vi "server_pos_indicator_v2.vi"(5 "reset":bool, 7 "rough":bool, 8 "error in":errorcluster, 10 "yc":dbl, 11 "xc":dbl) -> (0 "error out":errorcluster)   [LabVIEW 2014]
panel:
  out "resulting string":string
  out "rough Array":bool[](array[boolean])
  out "rough_num":i32
  out "size(s)":i32
  out "output array":T1(array[cluster])
  out "position":picture
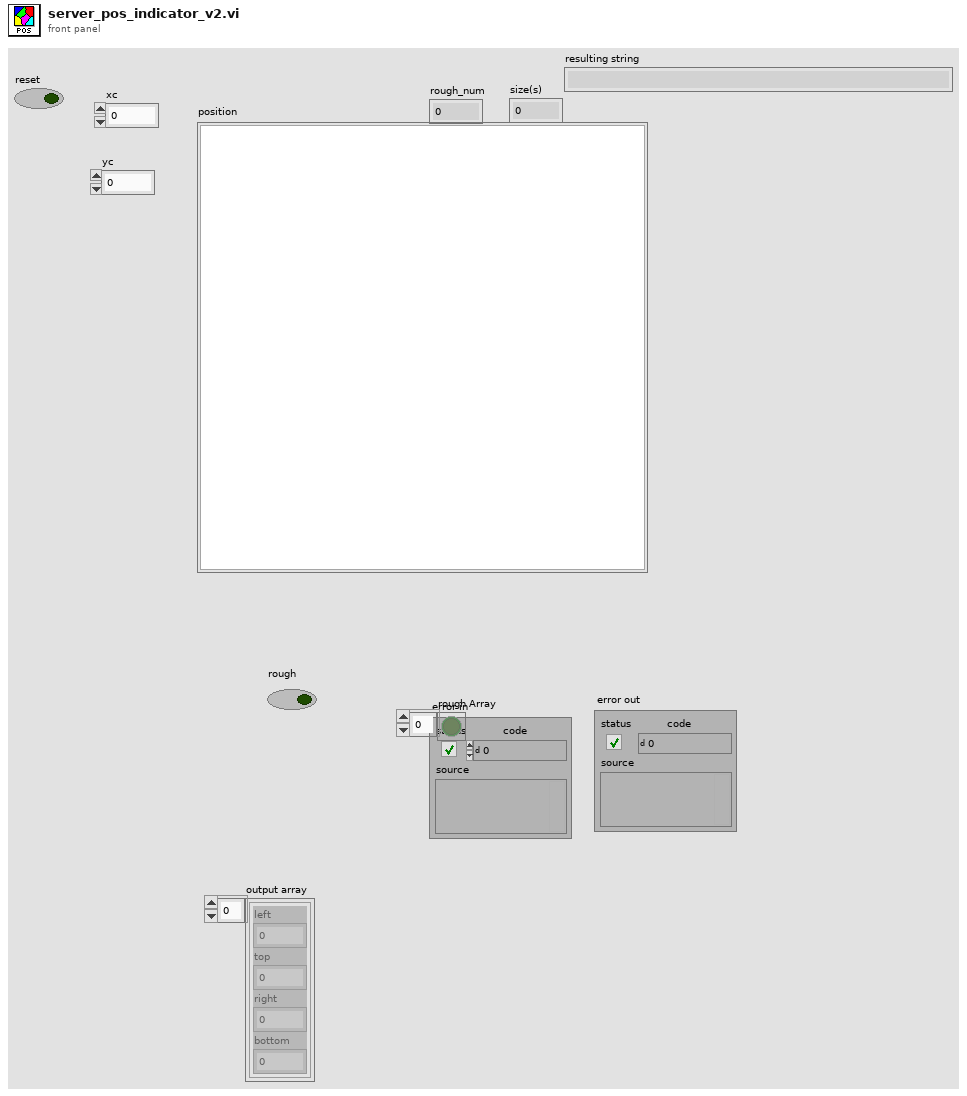
[diagram p1: front panel]
types:
  T1 = cluster{"left":i16, "top":i16, "right":i16, "bottom":i16}[]
  T2 = cluster{"left":i16, "top":i16, "right":i16, "bottom":i16}
  T3 = cluster{"horizontal":enum16{"left", "center", "right"}, "vertical":enum16{"top", "center", "bottom"}}
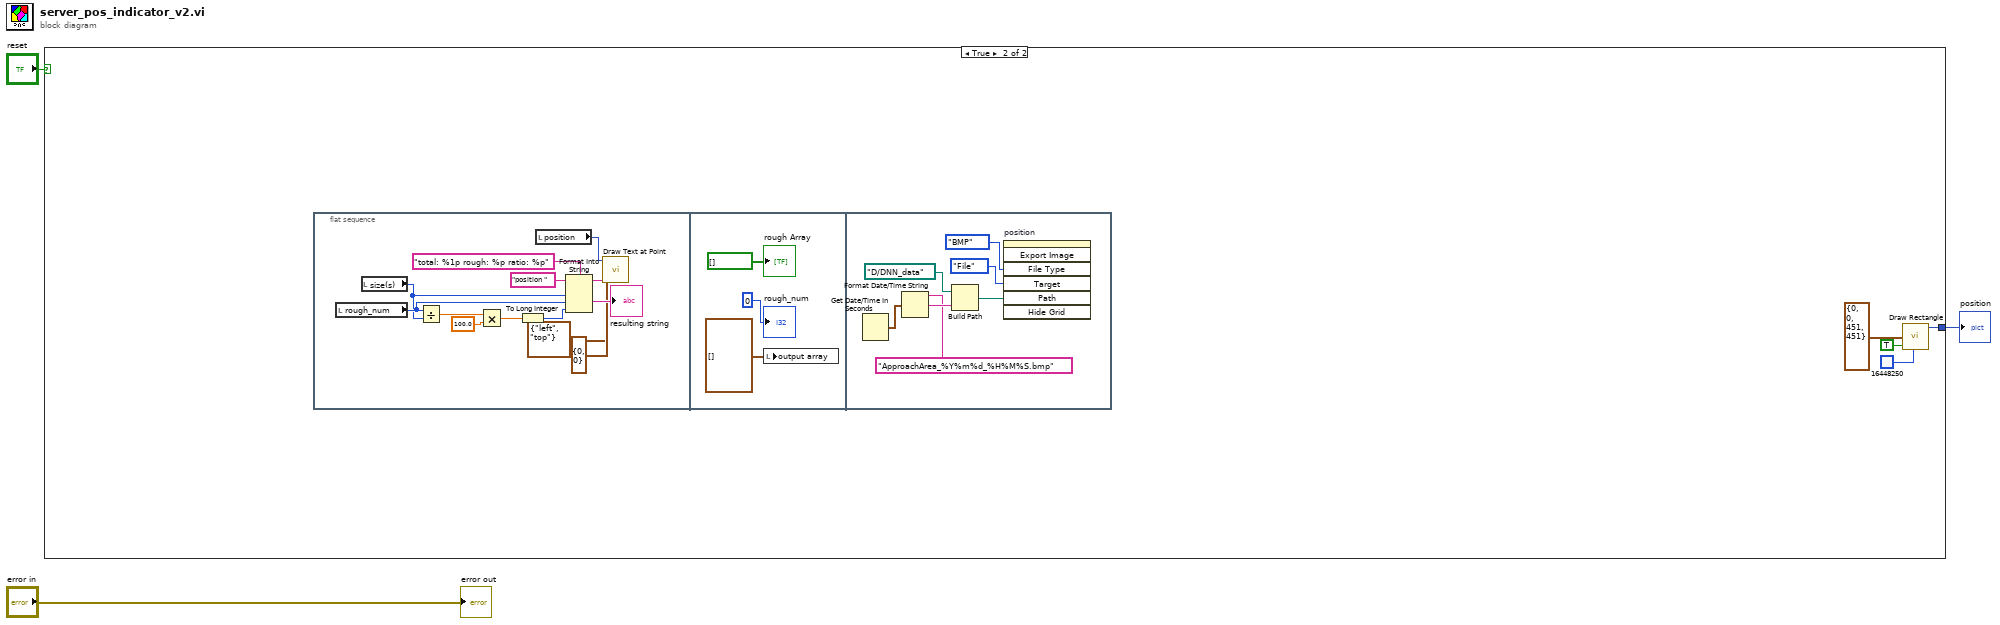
[diagram p0: block diagram]
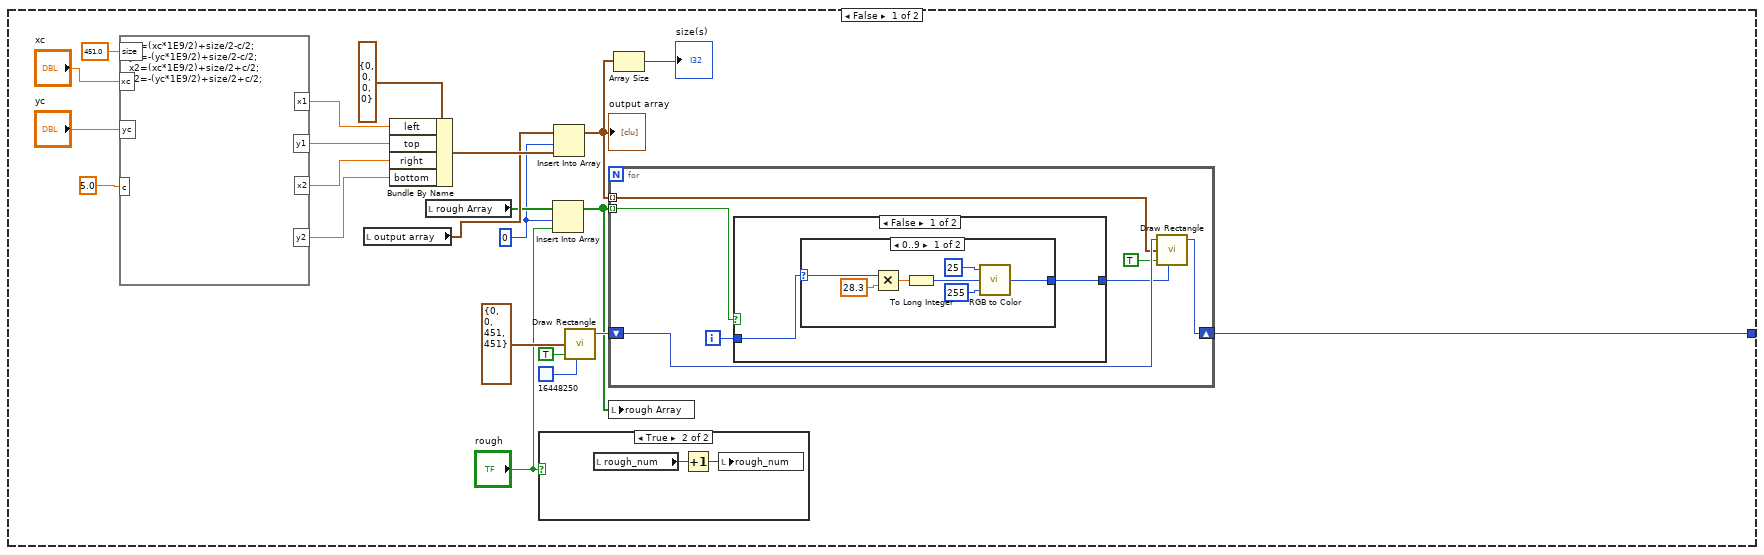
[diagram p2: hidden frame]
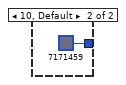
[diagram p4: hidden frame]
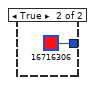
[diagram p5: hidden frame]
diagram:
  n1 = case shown="True" "reset" {
    tunnel: [w22 w46] -> w2
    frame False {
      w4 = 0 ("index")
      n2 = formula code="x1=(xc*1E9/2)+size/2-c/2;\ny1=-(yc*1E9/2)+size/2-c/2;\nx2=(xc*1E9/2)+size/2+c/2;\ny2=-(yc*1E9/2)+size/2+c/2;"("xc"="xc", "yc"="yc", "c"=5.0 ("input variable"), "size"=451.0 ("input variable")) -> ("x1"=w19:dbl, "y1"=w18:dbl, "x2"=w17:dbl, "y2"=w16:dbl)
      n3 = local read "output array"() -> (w8:T1)
      n4 = Bundle By Name(cluster=T2 {"left"=0, "top"=0, "right"=0, "bottom"=0} ("rect"), "left"=w19, "top"=w18, "right"=w17, "bottom"=w16) -> (w11:T2)
      n5 = local read "rough Array"() -> (w7:bool[])
      n6 = case shown="True" "rough" {
        frame False {
        }
        frame True {
          n7 = local read "rough_num"() -> (w27:i32)
          n8 = Increment(x=w27) -> (x+1=w26:i32)
          n9 = local write "rough_num"(w26) -> ()
        }
      }
      n10 = Insert Into Array(array=w7, index=w4, new element="rough") -> (w6:bool[])
      n11 = Insert Into Array(array=w8, index=w4, new element=w11) -> (w10:T1)
      "output array" <- w10
      n12 = call <vilib>:"Draw Rectangle.vi"("rect"=T2 {"left"=0, "top"=0, "right"=451, "bottom"=451}, "fill?(F)"=TRUE, "color(black)"=u32 16448250) -> ("new picture"=w24:picture)  [unwired: 6 in]
      n13 = for {
        shift-right: [w33] -> w22
        shift-left: w24 -> [w34]
        tunnel: w10 -> [w32] mode=indexing
        tunnel: w6 -> [w28] mode=indexing
        i -> [w31]
        n14 = case shown="False" w28 {
          tunnel: w31 -> [w36 _]
          tunnel: [w35 u32 16716306 ("color(black)")] -> w29
          frame False {
            n15 = case shown="0..9" w36 {
              selector: w36 -> [w40 _]
              tunnel: [w43 u32 7171459 ("color(black)")] -> w35
              frame 0..9 {
                n16 = Multiply(x=w40, y=28.3) -> (x*y=w42:dbl)
                n17 = To Long Integer(number=w42) -> (32bit integer=w41:i32)
                n18 = call <vilib>:"RGB to Color.vi"("B"=u8 255 ("R"), "G"=w41, "R"=u8 25 ("B")) -> ("Color"=w43:u32)
              }
              frame 10, Default {
              }
            }
          }
          frame True {
          }
        }
        n19 = call <vilib>:"Draw Rectangle.vi"("picture"=w34, "rect"=w32, "fill?(F)"=TRUE, "color(black)"=w29) -> ("new picture"=w33:picture)  [unwired: 5 in]
      }
      n20 = local write "rough Array"(w6) -> ()
      n21 = Array Size(array=w10) -> (size(s)=→"size(s)":i32)
    }
    frame True {
      n22 = flat-sequence {
        frame #0 {
          n23 = local read "rough_num"() -> (w59:i32)
          n24 = local read "size(s)"() -> (w58:i32)
          n25 = Divide(x=w59, y=w58) -> (x/y=w57:dbl)
          n26 = Multiply(x=w57, y=100.0) -> (x*y=w55:dbl)
          n27 = To Long Integer(number=w55) -> (32bit integer=w54:i32)
          n28 = local read "position"() -> (w53:picture)
          n29 = Format Into String(format string="total: %1p rough: %p ratio: %p", initial string="position ", w58, w59, w54) -> (resulting string=w52:string)  [unwired: 1 in, 1 out]
          "resulting string" <- w52
          n30 = call <vilib>:"Draw Text at Point.vi"("text"=w52, "alignment(left, top)"=T3 {"horizontal"=enum."left", "vertical"=enum."top"}, "origin"=cluster{"x":i16, "y":i16} {"x"=0, "y"=0}, "picture"=w53) -> ()  [unwired: 6 in, 2 out]
        }
        frame #1 {
          n31 = local write "output array"(T1 [] ("output array")) -> ()
          "rough_num" <- 0 ("rough")
          "rough Array" <- bool[] []
        }
        frame #2 {
          n32 = Get Date/Time In Seconds() -> (seconds since 1Jan1904=w66:timestamp)
          n33 = Format Date/Time String(time format string (%c)="ApproachArea_%Y%m%d_%H%M%S.bmp", seconds (now)=w66) -> (date/time string=w67:string)  [unwired: 1 in]
          n34 = Build Path(base path=path "D:/DNN_data" ("Path"), name or relative path=w67) -> (appended path=w71:path)
          n35 = invoke on="position" class="Pict" method="Export Image"("File Type"=enum32{"BMP", "EPS", "EMF", "PICT"}."BMP", "Target"=enum32{"File", "Clipboard"}."File", "Path"=w71) -> ()  [unwired: 4 in, 7 out]
        }
      }
      n36 = call <vilib>:"Draw Rectangle.vi"("rect"=T2 {"left"=0, "top"=0, "right"=451, "bottom"=451}, "fill?(F)"=TRUE, "color(black)"=u32 16448250) -> ("new picture"=w46:picture)  [unwired: 6 in]
    }
  }
  "position" <- w2
  "error out" <- "error in"
